vi "Python_ShowFrame.vi"() -> ()   [LabVIEW 2021]
doc: "This example demonstrates how to call a Python function and pass integers as arguments. It uses a python function to compute the sum of two integers."
panel:
  in  "session in":refnum<k35>
  in  "module path":path
  out "error out":errorcluster
  in  "error in (no error)":errorcluster
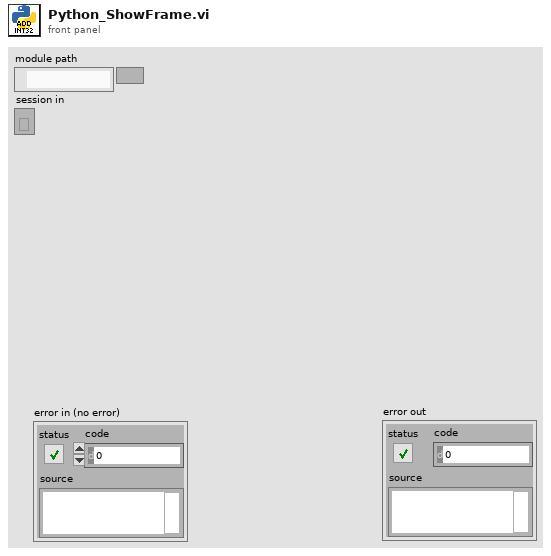
[diagram p1: front panel]
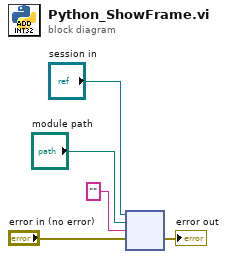
[diagram p0: block diagram]
diagram:
  n1 = node("session in", "module path", "" ("function name"), "error in (no error)") -> (→"error out":errorcluster)  [unwired: 2 in, 3 out]
